vi "SharedVariableMaster.vi"() -> ()   [LabVIEW 2014]
panel:
  out "threshold 3":i32
  out "name 8":string
  out "threshold 2":i32
  out "name 7":string
  out "threshold":i32
  out "name 6":string
  out "switch 5":i32
  out "name 5":string
  out "switch 4":i32
  out "name 4":string
  out "switch 3":i32
  out "name 3":string
  out "switch 2":i32
  out "name 2":string
  out "switch":i32
  out "name":string
  in  "Outlet5_Input":bool
  out "Outlet5_Output":bool
  in  "Outlet4_Input":bool
  out "Outlet4_Output":bool
  in  "Outlet3_Input":bool
  out "Outlet3_Output":bool
  in  "Outlet5_Refnum":refnum<k21>="ni.var.psp://Deepak-PC/Shared Variable Library Master/Outlet5"
  in  "Outlet3_Refnum":refnum<k21>="ni.var.psp://Deepak-PC/Shared Variable Library Master/Outlet3"
  in  "Outlet4_Refnum":refnum<k21>="ni.var.psp://Deepak-PC/Shared Variable Library Master/Outlet4"
  in  "Outlet2_Refnum":refnum<k21>="ni.var.psp://Deepak-PC/Shared Variable Library Master/Outlet2"
  out "Outlet2_Output":bool
  in  "Outlet2_Input":bool
  out "Outlet1_Output":bool
  in  "Outlet1_Input":bool
  in  "Outlet1_Refnum":refnum<k21>="ni.var.psp://Deepak-PC/Shared Variable Library Master/Outlet1"
  in  "Stop":bool
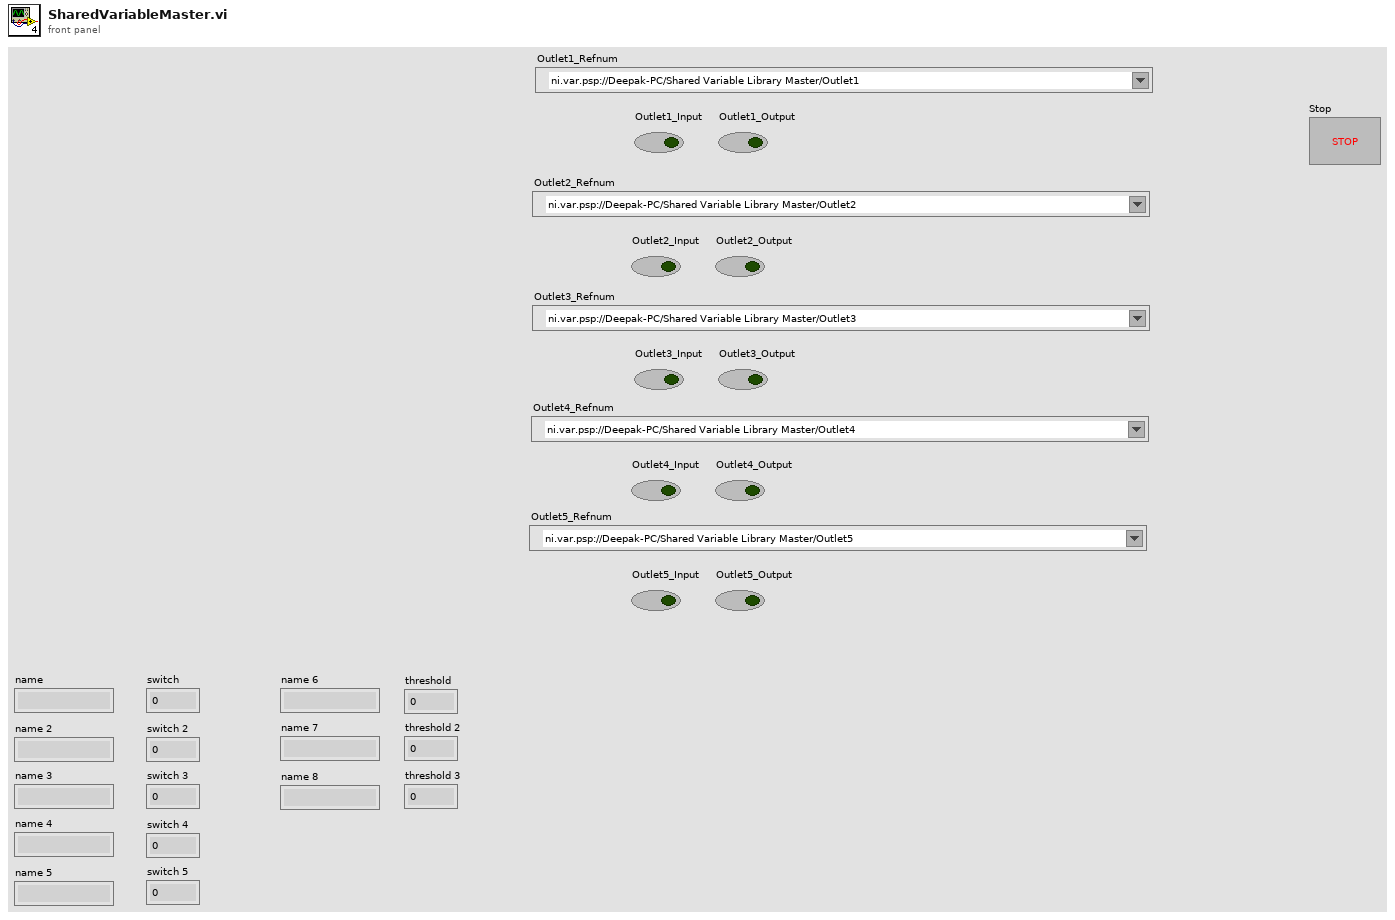
[diagram p1: front panel]
types:
  T1 = cluster{"[0]":cluster{"name":string, "switch":i32}, "[1]":cluster{"name":string, "switch":i32}, "[2]":cluster{"name":string, "switch":i32}, "[3]":cluster{"name":string, "switch":i32}, "[4]":cluster{"name":string, "switch":i32}, "[5]":cluster{"name":string, "switch":i32}, "[6]":cluster{"name":string, "switch":i32}, "[7]":cluster{"name":string, "switch":i32}, "[8]":cluster{"name":string, "switch":i32}}
  T2 = cluster{"[0]":cluster{"name":string, "threshold":i32}, "[1]":cluster{"name":string, "threshold":i32}, "[2]":cluster{"name":string, "threshold":i32}, "[3]":cluster{"name":string, "threshold":i32}, "[4]":cluster{"name":string, "threshold":i32}, "[5]":cluster{"name":string, "threshold":i32}, "[6]":cluster{"name":string, "threshold":i32}, "[7]":cluster{"name":string, "threshold":i32}, "[8]":cluster{"name":string, "threshold":i32}}
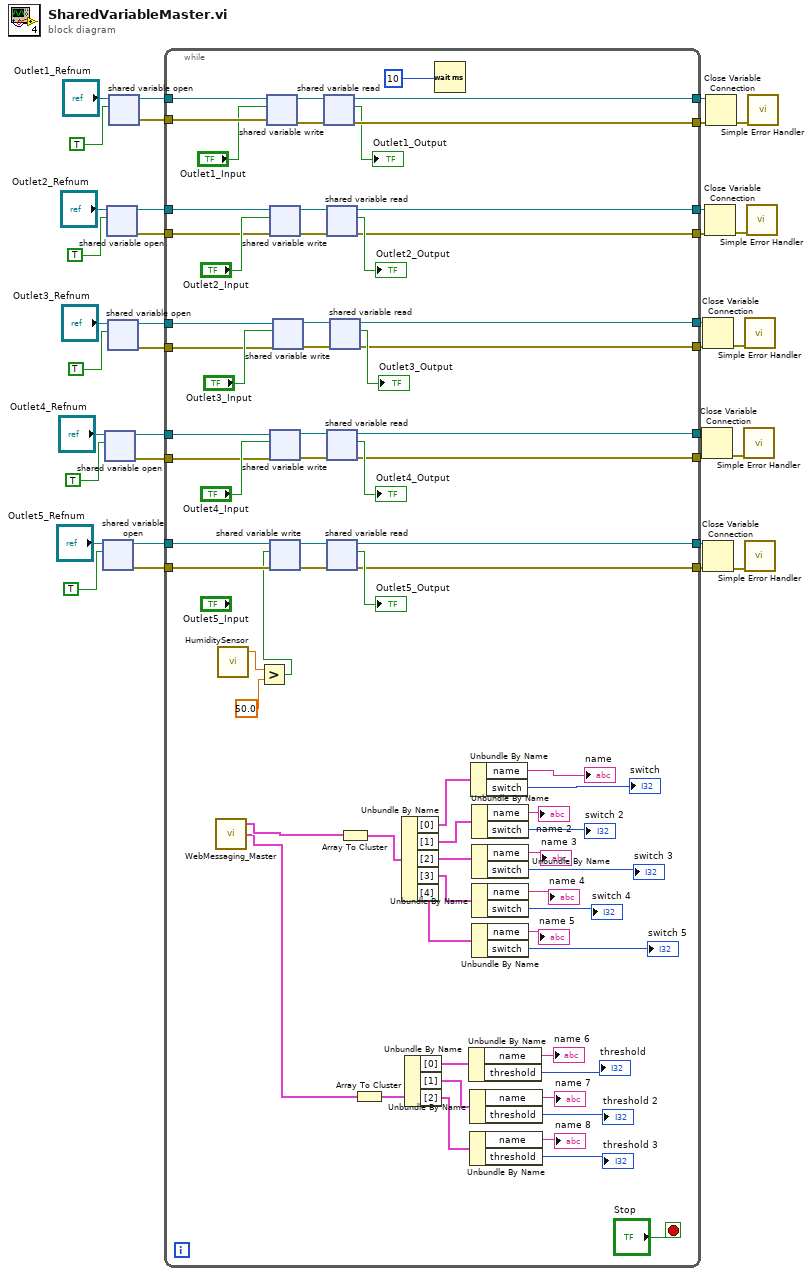
[diagram p0: block diagram]
diagram:
  n1 = shared-variable-open("Outlet5_Refnum", TRUE) -> (w4:refnum<k21>, w2:errorcluster)  [unwired: 2 in]
  n2 = shared-variable-open("Outlet4_Refnum", TRUE) -> (w8:refnum<k21>, w7:errorcluster)  [unwired: 2 in]
  n3 = shared-variable-open("Outlet2_Refnum", TRUE) -> (w25:refnum<k21>, w24:errorcluster)  [unwired: 2 in]
  n4 = shared-variable-open("Outlet3_Refnum", TRUE) -> (w12:refnum<k21>, w11:errorcluster)  [unwired: 2 in]
  n5 = shared-variable-open("Outlet1_Refnum", TRUE) -> (w32:refnum<k21>, w31:errorcluster)  [unwired: 2 in]
  n6 = while {
    tunnel: w32 -> [w103]
    tunnel: w31 -> [w102]
    tunnel: [w101] -> w30
    tunnel: [w100] -> w29
    tunnel: w25 -> [w93]
    tunnel: w24 -> [w92]
    tunnel: [w91] -> w23
    tunnel: [w90] -> w22
    tunnel: w12 -> [w78]
    tunnel: w11 -> [w77]
    tunnel: [w76] -> w10
    tunnel: [w75] -> w9
    tunnel: w8 -> [w74]
    tunnel: w7 -> [w73]
    tunnel: [w72] -> w6
    tunnel: [w71] -> w5
    tunnel: w4 -> [w70]
    tunnel: [w69] -> w3
    tunnel: w2 -> [w68]
    tunnel: [w67] -> w1
    stop <- "Stop" stop-if-true
    n7 = call "WebMessaging_Master.vi"() -> (1:w36:cluster{"name":string, "threshold":i32}[], 2:w37:cluster{"name":string, "switch":i32}[])  [unwired: 1 in]
    n8 = call "HumiditySensor.vi"() -> ("Humidity Waveform"=w64:dbl)  [unwired: 2 in]
    n9 = Greater?(x=w64, y=50.0) -> (0:w65:bool)
    n10 = shared-variable-write(w103, w102, "Outlet1_Input") -> (w105:refnum<k21>, w104:errorcluster)
    n11 = shared-variable-write(w93, w92, "Outlet2_Input") -> (w94:refnum<k21>, w95:errorcluster)
    n12 = shared-variable-write(w74, w73, "Outlet4_Input") -> (w82:refnum<k21>, w83:errorcluster)
    n13 = shared-variable-write(w70, w68, w65) -> (w81:refnum<k21>, w80:errorcluster)
    n14 = shared-variable-write(w78, w77, "Outlet3_Input") -> (w89:refnum<k21>, w88:errorcluster)
    n15 = shared-variable-read(w105, w104) -> (w101:refnum<k21>, w100:errorcluster, →"Outlet1_Output":bool)  [unwired: 1 out]
    n16 = shared-variable-read(w94, w95) -> (w91:refnum<k21>, w90:errorcluster, →"Outlet2_Output":bool)  [unwired: 1 out]
    n17 = shared-variable-read(w82, w83) -> (w72:refnum<k21>, w71:errorcluster, →"Outlet4_Output":bool)  [unwired: 1 out]
    n18 = shared-variable-read(w81, w80) -> (w69:refnum<k21>, w67:errorcluster, →"Outlet5_Output":bool)  [unwired: 1 out]
    n19 = shared-variable-read(w89, w88) -> (w76:refnum<k21>, w75:errorcluster, →"Outlet3_Output":bool)  [unwired: 1 out]
    n20 = Array To Cluster(array=w37) -> (cluster=w63:T1)
    n21 = Array To Cluster(array=w36) -> (cluster=w47:T2)
    n22 = Unbundle By Name(w63) -> ("[0]"=w62:cluster{"name":string, "switch":i32}, "[1]"=w61:cluster{"name":string, "switch":i32}, "[2]"=w60:cluster{"name":string, "switch":i32}, "[3]"=w59:cluster{"name":string, "switch":i32}, "[4]"=w58:cluster{"name":string, "switch":i32})
    n23 = Unbundle By Name(w47) -> ("[0]"=w46:cluster{"name":string, "threshold":i32}, "[1]"=w45:cluster{"name":string, "threshold":i32}, "[2]"=w44:cluster{"name":string, "threshold":i32})
    n24 = Wait (ms)(milliseconds to wait=u32 10 ("millisecond timer value")) -> ()  [unwired: 1 out]
    n25 = Unbundle By Name(w46) -> ("name"=→"name 6":string, "threshold"=→"threshold":i32)
    n26 = Unbundle By Name(w45) -> ("name"=→"name 7":string, "threshold"=→"threshold 2":i32)
    n27 = Unbundle By Name(w44) -> ("name"=→"name 8":string, "threshold"=→"threshold 3":i32)
    n28 = Unbundle By Name(w62) -> ("name"=→"name":string, "switch"=→"switch":i32)
    n29 = Unbundle By Name(w61) -> ("name"=→"name 2":string, "switch"=→"switch 2":i32)
    n30 = Unbundle By Name(w60) -> ("name"=→"name 3":string, "switch"=→"switch 3":i32)
    n31 = Unbundle By Name(w59) -> ("name"=→"name 4":string, "switch"=→"switch 4":i32)
    n32 = Unbundle By Name(w58) -> ("name"=→"name 5":string, "switch"=→"switch 5":i32)
  }
  n33 = Close Variable Connection(8:w5, 11:w6) -> (0:w15:errorcluster)
  n34 = Close Variable Connection(8:w9, 11:w10) -> (0:w14:errorcluster)
  n35 = Close Variable Connection(8:w1, 11:w3) -> (0:w13:errorcluster)
  n36 = Close Variable Connection(8:w22, 11:w23) -> (0:w26:errorcluster)
  n37 = Close Variable Connection(8:w29, 11:w30) -> (0:w33:errorcluster)
  n38 = call <vilib>:"Simple Error Handler.vi"("error in (no error)"=w15) -> ()  [unwired: 4 in, 5 out]
  n39 = call <vilib>:"Simple Error Handler.vi"("error in (no error)"=w14) -> ()  [unwired: 4 in, 5 out]
  n40 = call <vilib>:"Simple Error Handler.vi"("error in (no error)"=w13) -> ()  [unwired: 4 in, 5 out]
  n41 = call <vilib>:"Simple Error Handler.vi"("error in (no error)"=w26) -> ()  [unwired: 4 in, 5 out]
  n42 = call <vilib>:"Simple Error Handler.vi"("error in (no error)"=w33) -> ()  [unwired: 4 in, 5 out]
